vi "calibrar.vi"(2 "V 2":dbl, 3 "V1":dbl, 4 "Temp2":dbl, 5 "Temp":dbl) -> (0 "B":dbl, 1 "A":dbl)   [LabVIEW 2014]
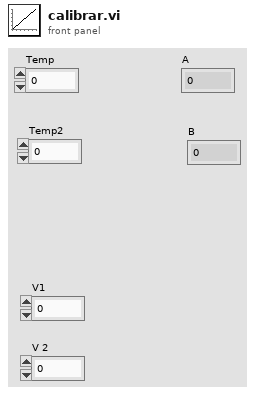
[diagram p1: front panel]
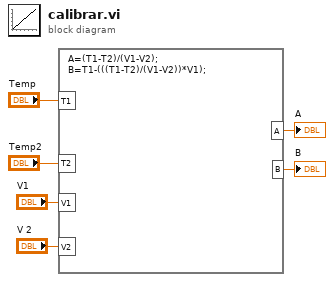
[diagram p0: block diagram]
diagram:
  n1 = formula code="A=(T1-T2)/(V1-V2);\nB=T1-(((T1-T2)/(V1-V2))*V1);"("T1"="Temp", "T2"="Temp2", "V1"="V1", "V2"="V 2") -> ("A"=→"A":dbl, "B"=→"B":dbl)
